vi "readADC.vi"(7 "x(0), y(0)":fxp<+/-,16,5>[](array[numeric]), 8 "z-height":refnum<k21>="Mod2/AI0", 9 "z-err- ADC":refnum<k21>="Mod2/AI0", 10 "y - ADC":refnum<k21>="Mod2/AI0", 11 "x - ADC":refnum<k21>="Mod2/AI0") -> (2 "x_y_ze_z_k":fxp<+/-,25,6>[](array[numeric]))   [LabVIEW 2017]
uses:
  <vilib>/rvi/eio/common/nirviEmuTemplateMethod_errors.vi
  <vilib>/eio/EIONode/EIONode.xnode
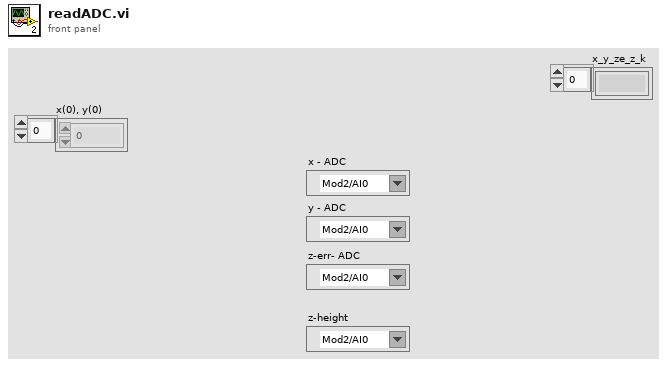
[diagram p1: front panel]
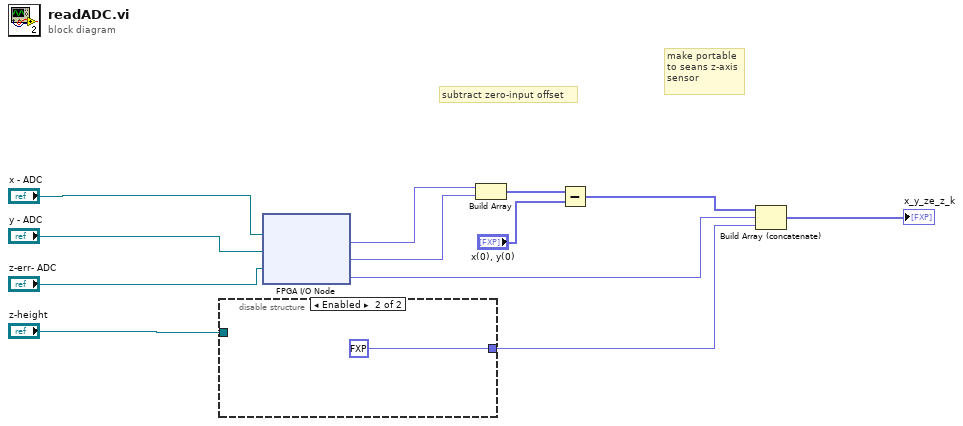
[diagram p0: block diagram]
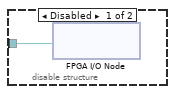
[diagram p2: hidden frame]
diagram:
  # "make portable\nto seans z-axis\nsensor"
  # "subtract zero-input offset"
  n1 = disable-structure shown="Enabled" {
    disable-tunnel: "z-height" -> [w13 _]
    disable-tunnel: [_ fxp<+,1,1> 0.0] -> w1
    frame Disabled {
      n2 = xnode "FPGA I/O Node"("FPGA I/O In"=w13) -> ()  [unwired: 2 out]
    }
    frame Enabled {
    }
  }
  n3 = xnode "FPGA I/O Node"("FPGA I/O In"="x - ADC", "FPGA I/O In"="y - ADC", "FPGA I/O In"="z-err- ADC") -> ("I/O Item"=w10:fxp<+/-,24,5>, "I/O Item"=w4:fxp<+/-,24,5>, "I/O Item"=w12:fxp<+/-,24,5>)  [unwired: 3 out]
  n4 = Build Array(w10, w4) -> (w9:fxp<+/-,24,5>[])
  n5 = Subtract(x=w9, y="x(0), y(0)") -> (x-y=w7:fxp<+/-,25,6>[])
  n6 = Build Array (concatenate)(w7, w12, w1) -> (→"x_y_ze_z_k":fxp<+/-,25,6>[])
